vi "Load Transition Config.vi"(8 "error in (no error)":errorcluster, 10 "Config Element":refnum<class "Config Element.lvclass">, 11 "State Transition Config in":refnum<class "State Transition Config.lvclass">) -> (0 "error out":errorcluster, 3 "State Transition Config out":refnum<class "State Transition Config.lvclass">)   [LabVIEW 2020, in "VolatusSeqConfig.lvlib" / "State Transition Config.lvclass"]
uses:
  State Transition Config.lvclass
  State Transition Config.lvclass/State Transition Config.ctl
  lv-cdm/CDM-Config/Config Element/Config Element.lvclass
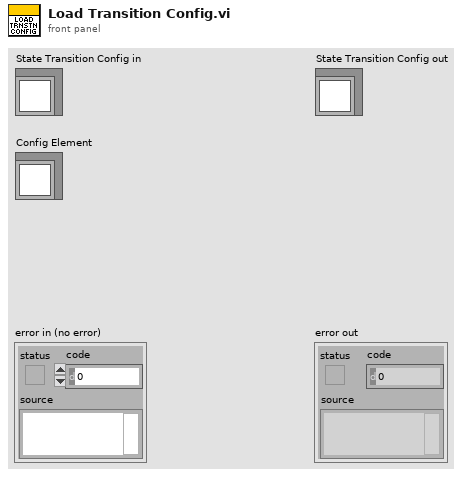
[diagram p1: front panel]
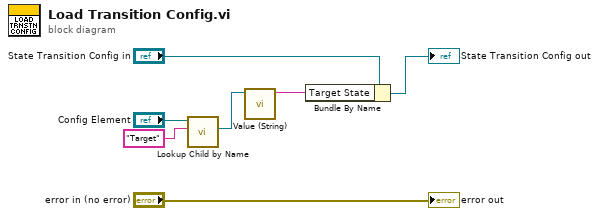
[diagram p0: block diagram]
diagram:
  n1 = call "Lookup Child by Name.vi"("Name"="Target", "Config Element in"="Config Element") -> ("Child"=w3:refnum<class "Config Element.lvclass">)  [unwired: 6 in, 3 out]
  n2 = call "Value (String).vi"("Config Element in"=w3) -> ("String Value"=w1:string)  [unwired: 9 in, 1 out]
  n3 = Bundle By Name(cluster="State Transition Config in", "Target State"=w1) -> (→"State Transition Config out":refnum<class "State Transition Config.lvclass">)
  "error out" <- "error in (no error)"
